vi "add mapping.vi"(7 "owner ID":string, 8 "error in":errorcluster, 9 "action channel":refnum<class "TBM channel.lvclass">, 10 "seq channel":refnum<class "TBM channel.lvclass">, 11 "engine configuration":refnum<class "base TBM sequencer configuration.lvclass">) -> (0 "error out":errorcluster, 3 "engine configuration out":refnum<class "base TBM sequencer configuration.lvclass">)   [LabVIEW 2014, in "base TBM sequencer configuration.lvclass"]
uses:
  base TBM sequencer configuration.lvclass
  <vilib>/NI/Tag Bus Module Framework/channel/TBM channel.lvclass
  <vilib>/NI/Tag Bus/tag/tag descriptor.lvclass/tag descriptor.ctl
  <vilib>/NI/Tag Bus Module Framework/channel/TBM channel.lvclass/TBM channel.ctl
  base TBM sequencer configuration.lvclass/base TBM sequencer configuration.ctl
  Module Mappings.ctl
  <vilib>/NI/Tag Bus/table/mapping specification.ctl
  <vilib>/NI/Tag Bus/tag/Data Type.ctl
  <vilib>/NI/Tag Bus/table/mapping.ctl
  <vilib>/NI/Tag Bus/tag/read tag name.vi
  <vilib>/NI/Tag Bus Module Framework/channel/Read channel classification.vi
  <vilib>/NI/Tag Bus/tag/read data type.vi
  <vilib>/NI/Tag Bus/tag/tag descriptor.lvclass
  <vilib>/NI/Tag Bus/table/data table.lvlib
  <vilib>/NI/Configuration Framework/NISE_CEF_TreeControl.lvlib
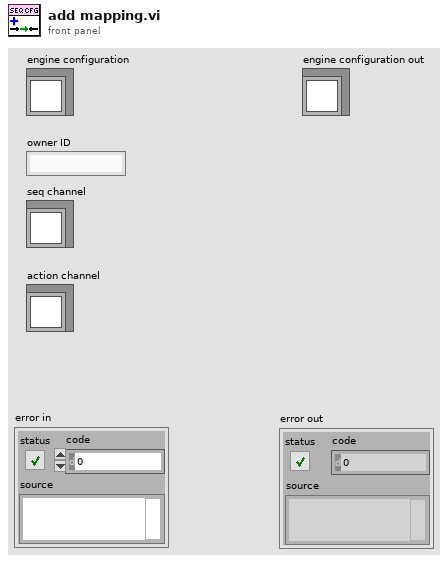
[diagram p1: front panel]
types:
  T1 = typedef "base TBM sequencer configuration.lvclass/Module Mappings.ctl" = cluster{"Owning ID":string, "Input Mappings":T2[], "Process Parameter Mappings":T2[], "Process Results Mappings":T2[], "Output Mappings":T2[]}
  T2 = typedef "tag bus.lvlib/data table.lvlib/mapping specification.ctl" = cluster{"data type":T3, "mappings":T4[]}
  T3 = typedef "tag bus.lvlib/tag descriptor.lvclass/Data Type.ctl" = enum16{"Double", "Single", "I64", "I32", "I16", "I8", "U64", "U32", "U16", "U8", "Boolean", "String", "Array of Double", "Array of Single", "Array of I64", "Array of I32", "Array of I16", "Array of I8", "Array of U64", "Array of U32", "Array of U16", "Array of U8", "Array of Boolean", "Array of String"}
  T4 = typedef "tag bus.lvlib/data table.lvlib/mapping.ctl" = cluster{"sink name":string, "source name":string}
  T5 = typedef "TBM channel.lvclass/channel classification.ctl" = enum16{"input data", "output data", "processing parameter", "processing result"}
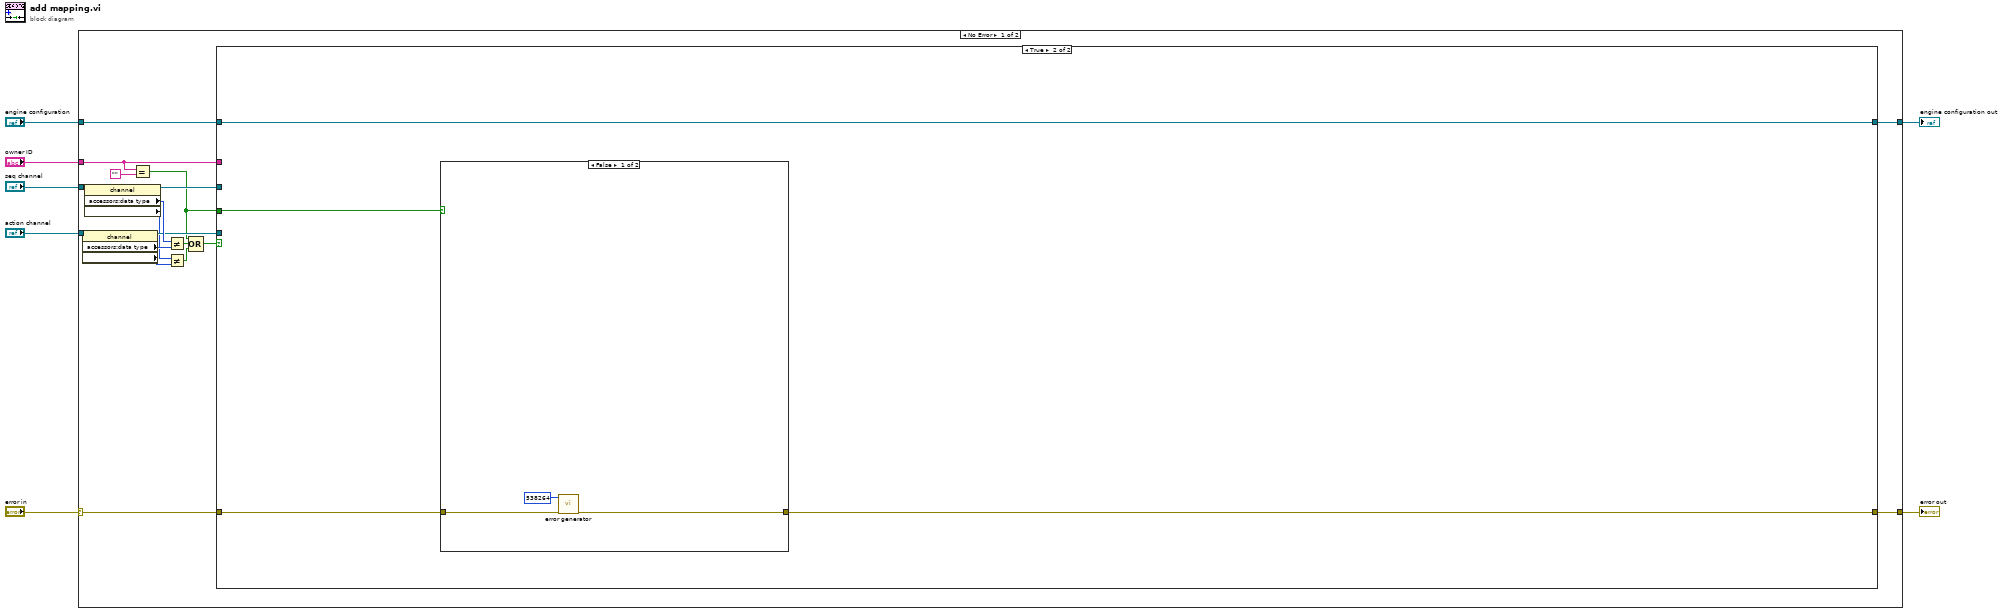
[diagram p0: block diagram]
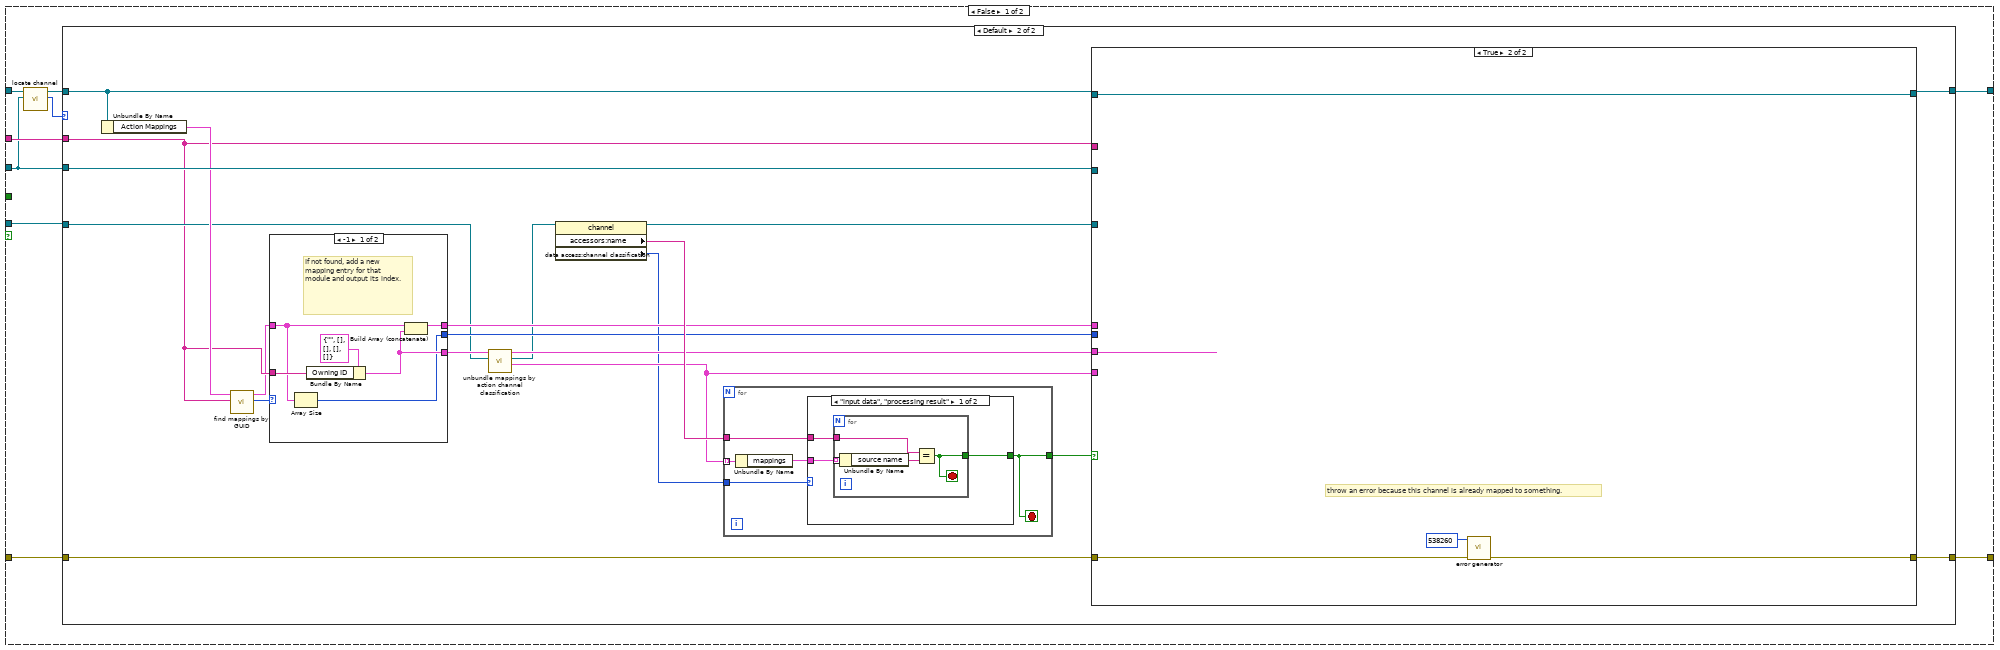
[diagram p2: hidden frame]
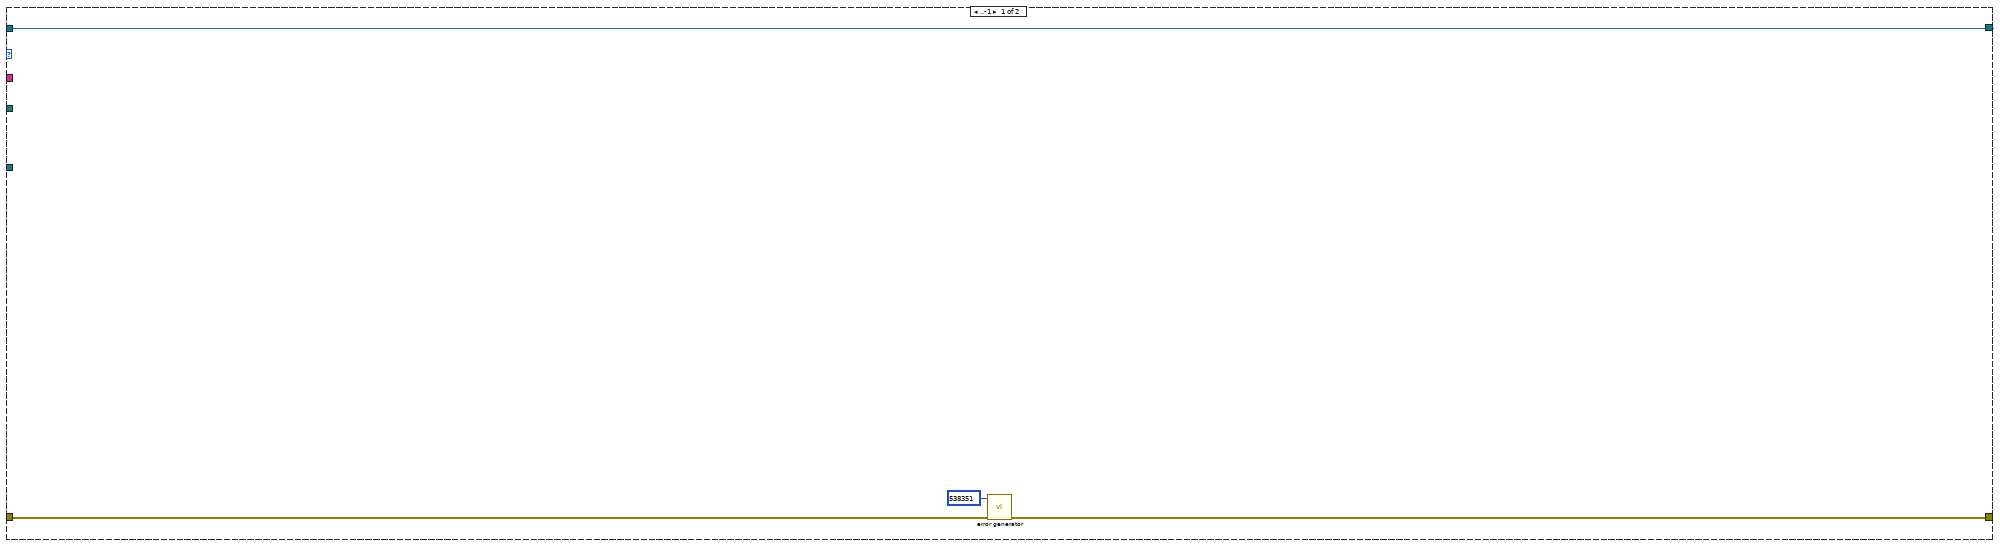
[diagram p3: hidden frame]
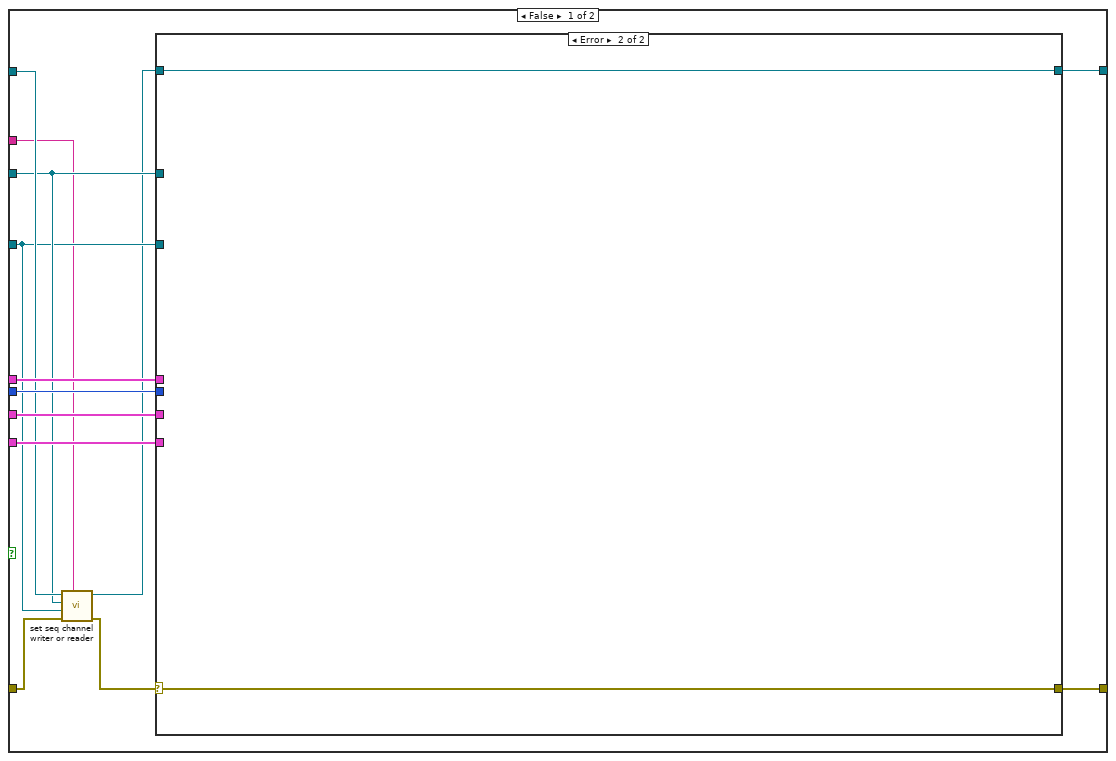
[diagram p4: hidden frame]
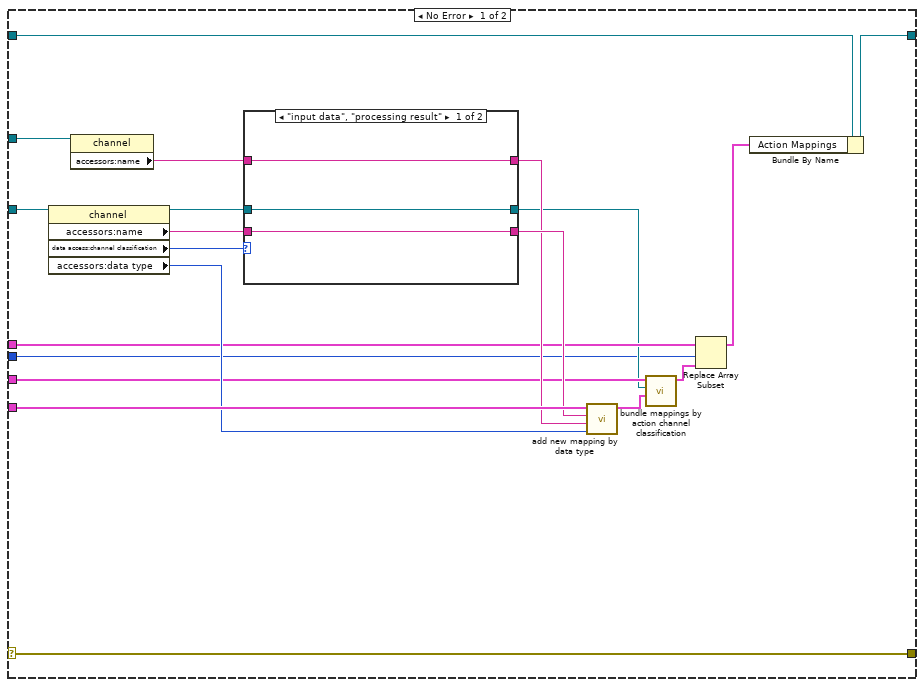
[diagram p5: hidden frame]
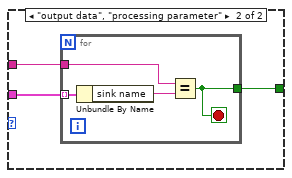
[diagram p7: hidden frame]
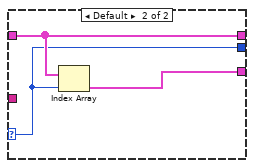
[diagram p8: hidden frame]
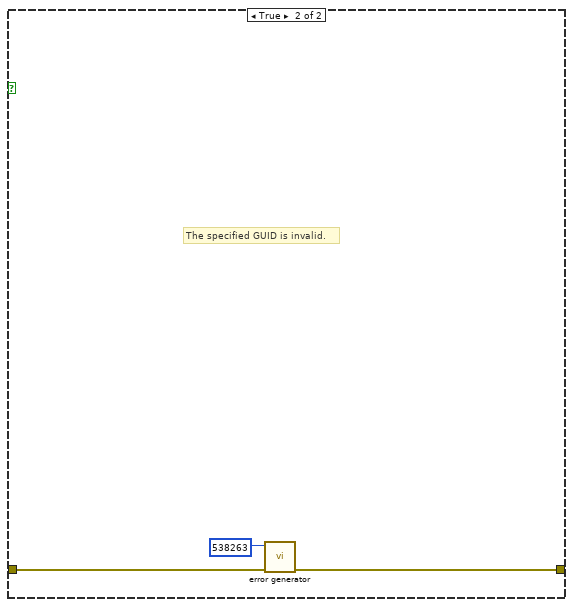
[diagram p9: hidden frame]
diagram:
  n1 = case shown="No Error" "error in" {
    selector: "error in" -> [w20 w142]
    tunnel: "owner ID" -> [w12 _]
    tunnel: "engine configuration" -> [w16 w143]
    tunnel: "seq channel" -> [w25 _]
    tunnel: "action channel" -> [w24 _]
    tunnel: [w21 w143] -> w3
    tunnel: [w19 w142] -> w1
    frame No Error {
      n2 = property class="channel"(reference=w24) -> (reference out=w18:refnum<class "TBM channel.lvclass">, "accessors:data type"=w23:T3, "data access:channel classification"=w8:T5)  [unwired: 1 in, 1 out]
      n3 = property class="channel"(reference=w25) -> (reference out=w17:refnum<class "TBM channel.lvclass">, "accessors:data type"=w22:T3, "data access:channel classification"=w9:T5)  [unwired: 1 in, 1 out]
      n4 = Equal?(x=w12, y="") -> (x = y?=w11:bool)
      n5 = Not Equal?(x=w22, y=w23) -> (x != y?=w15:bool)
      n6 = Not Equal?(x=w9, y=w8) -> (x != y?=w10:bool)
      n7 = Compound Arithmetic op=OR(w11, w15, w10) -> (w14:bool)
      n8 = case shown="True" w14 {
        tunnel: w16 -> [w32 w135]
        tunnel: w12 -> [w34 _]
        tunnel: [w27 w135] -> w21
        tunnel: w20 -> [w28 w133]
        tunnel: [w26 w132] -> w19
        tunnel: w17 -> [w29 _]
        tunnel: w18 -> [w33 _]
        tunnel: w11 -> [_ w134]
        frame False {
          n9 = call "locate channel.vi"("tag descriptor"=w29, "sequencer config in"=w32) -> ("index"=w30:i32, "sequencer config out"=w31:refnum<class "base TBM sequencer configuration.lvclass">)  [unwired: 8 in]
          n10 = case shown="Default" w30 {
            tunnel: w34 -> [_ w40]
            tunnel: w31 -> [w38 w52]
            tunnel: w33 -> [_ w42]
            tunnel: w29 -> [_ w54]
            tunnel: w28 -> [w37 w56]
            tunnel: [w36 w53] -> w26
            tunnel: [w38 w51] -> w27
            frame ..-1 {
              n11 = call <vilib>:"error generator.vi"("error in"=w37, "error code (0)"=538351) -> ("error out"=w36:errorcluster)  [unwired: 7 in]
            }
            frame Default {
              n12 = Unbundle By Name(w52) -> ("Action Mappings"=w50:T1[])
              n13 = call "find mappings by GUID.vi"("owner ID"=w40, "action Mappings"=w50) -> ("index"=w49:i32, "action Mappings out"=w39:T1[])  [unwired: 8 in]
              n14 = case shown="-1" w49 {
                selector: w49 -> [_ w129]
                tunnel: w39 -> [w124 w131]
                tunnel: [w126 w131] -> w48
                tunnel: [w125 w130] -> w46
                tunnel: [w123 w129] -> w47
                tunnel: w40 -> [w127 _]
                frame -1 {
                  # "If not found, add a new mapping entry for that module and output its index."
                  n15 = Array Size(array=w124) -> (size(s)=w123:i32)
                  n16 = Bundle By Name(cluster=T1 {"Owning ID"="", "Input Mappings"=[], "Process Parameter Mappings"=[], "Process Results Mappings"=[], "Output Mappings"=[]} ("Component Mappings"), "Owning ID"=w127) -> (w125:T1)
                  n17 = Build Array (concatenate)(w124, w125) -> (w126:T1[])
                }
                frame Default {
                  n18 = Index Array(array=w131, index=w129) -> (element=w130:T1)
                }
              }
              n19 = call "unbundle mappings by action channel classification.vi"("channel"=w42, "Mappings"=w46) -> ("Mappings For One Method"=w45:T2[], "channel out"=w43:refnum<class "TBM channel.lvclass">, "Mappings out"=w44:T1)  [unwired: 7 in]
              n20 = property class="channel"(reference=w43) -> (reference out=w58:refnum<class "TBM channel.lvclass">, "accessors:name"=w57:string, "data access:channel classification"=w41:T5)  [unwired: 1 in, 1 out]
              n21 = for {
                tunnel: w45 -> [w108] mode=indexing
                tunnel: w41 -> [w107]
                tunnel: w57 -> [w105]
                tunnel: [w104] -> w55
                stop <- w104 stop-if-true
                n22 = Unbundle By Name(w108) -> ("mappings"=w106:T4[])
                n23 = case shown="\"input data\", \"processing result\"" w107 {
                  tunnel: w106 -> [w110 w118]
                  tunnel: w105 -> [w111 w117]
                  tunnel: [w109 w116] -> w104
                  frame "input data", "processing result" {
                    n24 = for {
                      tunnel: w110 -> [w115] mode=indexing
                      tunnel: w111 -> [w113]
                      tunnel: [w112] -> w109
                      stop <- w112 stop-if-true
                      n25 = Unbundle By Name(w115) -> ("source name"=w114:string)
                      n26 = Equal?(x=w113, y=w114) -> (x = y?=w112:bool)
                    }
                  }
                  frame "output data", "processing parameter" {
                    n27 = for {
                      tunnel: w118 -> [w122] mode=indexing
                      tunnel: w117 -> [w120]
                      tunnel: [w119] -> w116
                      stop <- w119 stop-if-true
                      n28 = Unbundle By Name(w122) -> ("sink name"=w121:string)
                      n29 = Equal?(x=w120, y=w121) -> (x = y?=w119:bool)
                    }
                  }
                }
              }
              n30 = case shown="True" w55 {
                tunnel: w58 -> [w63 _]
                tunnel: w45 -> [w71 _]
                tunnel: w56 -> [w66 w101]
                tunnel: w54 -> [w64 _]
                tunnel: [w60 w100] -> w53
                tunnel: w48 -> [w69 _]
                tunnel: w47 -> [w67 _]
                tunnel: w44 -> [w68 _]
                tunnel: w52 -> [w65 w103]
                tunnel: [w70 w103] -> w51
                tunnel: w40 -> [w62 _]
                frame False {
                  n31 = call "set seq channel writer or reader.vi"("module GUID"=w62, "error in"=w66, "channel"=w63, "tag descriptor"=w64, "sequencer config in"=w65) -> ("error out"=w61:errorcluster, "sequencer config out"=w59:refnum<class "base TBM sequencer configuration.lvclass">)  [unwired: 5 in]
                  n32 = case shown="Error" w61 {
                    selector: w61 -> [w73 w98]
                    tunnel: w71 -> [w90 _]
                    tunnel: [w83 w99] -> w70
                    tunnel: w69 -> [w81 _]
                    tunnel: w68 -> [w80 _]
                    tunnel: w67 -> [w76 _]
                    tunnel: w64 -> [w75 _]
                    tunnel: w63 -> [w74 _]
                    tunnel: [w73 w98] -> w60
                    tunnel: w59 -> [w72 w99]
                    frame No Error {
                      n33 = property class="channel"(reference=w74) -> (reference out=w82:refnum<class "TBM channel.lvclass">, "accessors:name"=w88:string, "data access:channel classification"=w85:T5, "accessors:data type"=w89:T3)  [unwired: 1 in, 1 out]
                      n34 = property class="channel"(reference=w75) -> ("accessors:name"=w91:string)  [unwired: 1 in, 2 out]
                      n35 = case shown="\"input data\", \"processing result\"" w85 {
                        tunnel: w88 -> [w93 w96]
                        tunnel: w91 -> [w94 w97]
                        tunnel: [w94 w96] -> w86
                        tunnel: [w93 w97] -> w87
                        tunnel: w82 -> [w92 w95]
                        tunnel: [w92 w95] -> w79
                        frame "input data", "processing result" {
                        }
                        frame "output data", "processing parameter" {
                        }
                      }
                      n36 = call "add new mapping by data type.vi"("data type"=w89, "sink name"=w86, "source name"=w87, "mappings"=w90) -> ("mappings out"=w78:T2[])  [unwired: 7 in]
                      n37 = call "bundle mappings by action channel classification.vi"("Mappings For One Method"=w78, "channel"=w79, "Mappings"=w80) -> ("Mappings out"=w77:T1)  [unwired: 7 in, 1 out]
                      n38 = Replace Array Subset(array=w81, new element=w77, index=w76) -> (w84:T1[])
                      n39 = Bundle By Name(cluster=w72, "Action Mappings"=w84) -> (w83:refnum<class "base TBM sequencer configuration.lvclass">)
                    }
                    frame Error {
                    }
                  }
                }
                frame True {
                  # "throw an error because this channel is already mapped to something."
                  n40 = call <vilib>:"error generator.vi"("error in"=w101, "error code (0)"=538260) -> ("error out"=w100:errorcluster)  [unwired: 7 in]
                }
              }
            }
          }
        }
        frame True {
          n41 = case shown="False" w134 {
            tunnel: w133 -> [w137 w140]
            tunnel: [w136 w139] -> w132
            frame False {
              n42 = call <vilib>:"error generator.vi"("error in"=w137, "error code (0)"=538264) -> ("error out"=w136:errorcluster)  [unwired: 7 in]
            }
            frame True {
              # "The specified GUID is invalid."
              n43 = call <vilib>:"error generator.vi"("error in"=w140, "error code (0)"=538263) -> ("error out"=w139:errorcluster)  [unwired: 7 in]
            }
          }
        }
      }
    }
    frame Error {
    }
  }
  "error out" <- w1
  "engine configuration out" <- w3
